vi "setFABroadcastCounter.vi"(10 "FABroadcastCounter":u8, 11 "ILCCommunications in":refnum<class "ILCCommunications.lvclass">) -> (3 "ILCCommunications out":refnum<class "ILCCommunications.lvclass">)   [LabVIEW 2016, in "ILCCommunications.lvclass"]
uses:
  ILCCommunications.lvclass
  ILCCommunications.lvclass/ILCCommunications.ctl
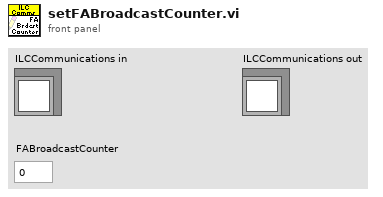
[diagram p1: front panel]
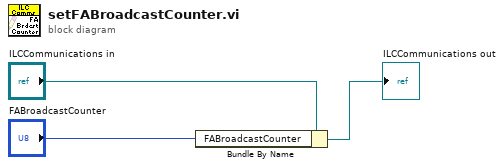
[diagram p0: block diagram]
diagram:
  n1 = Bundle By Name(cluster="ILCCommunications in", "FABroadcastCounter"="FABroadcastCounter") -> (→"ILCCommunications out":refnum<class "ILCCommunications.lvclass">)
